vi "closed hold.vi"(2 "Acrade Drive?":bool=TRUE, 3 "Y axis value (Left)":dbl, 4 "X axis value (Right)":dbl, 5 "Threshold (.4)":dbl=0.4) -> (0 "right":dbl format="%.2f", 1 "left":dbl format="%.2f")   [LabVIEW 2014]
doc: "Holds the drivetrain position, so the robot resists movement. This is useful when balancing bridges. It's like a software brake... This VI also allows for the driver to make slight adjustments in robot position."
uses:
  <vilib>/addons/control/pid/pid.llb/PID (DBL).vi
  <vilib>/addons/control/pid/NI_PID_pid.lvlib
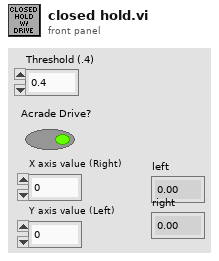
[diagram p1: front panel]
types:
  T1 = typedef "WPI_EncoderDevRef.ctl" = cluster{"DevStatus":errorcluster, "EncoderIndex":T2, "CounterIndex":T3, "DistancePerCount":dbl, "Decoding Type":T4}
  T2 = typedef "FPGA_EncoderIdx.ctl" = enum8{"Enc 0", "Enc 1", "Enc 2", "Enc 3", "Enc 4", "Enc 5", "Enc 6", "Enc 7", "Invalid"}
  T3 = typedef "FPGA_CounterCtrSystemIndex.ctl" = enum8{"Ctr 0", "Ctr 1", "Ctr 2", "Ctr 3", "Ctr 4", "Ctr 5", "Ctr 6", "Ctr 7", "Invalid"}
  T4 = typedef "WPI_EncoderType.ctl" = enum16{"1x", "2x", "4x"}
  T5 = cluster{"proportional gain (Kc)":dbl, "integral time (Ti, min)":dbl, "derivative time (Td, min)":dbl}
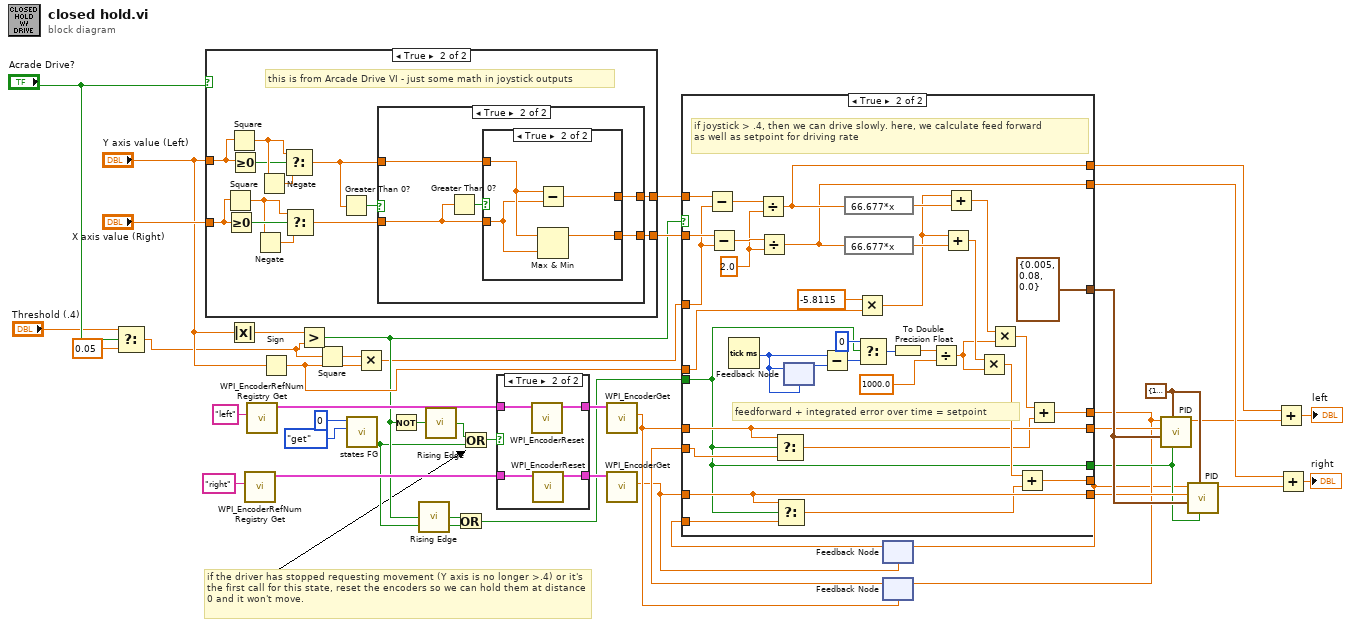
[diagram p0: block diagram]
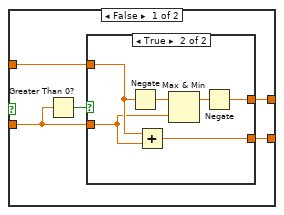
[diagram p3: hidden frame]
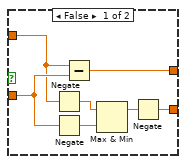
[diagram p4: hidden frame]
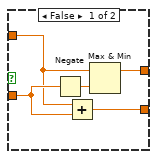
[diagram p5: hidden frame]
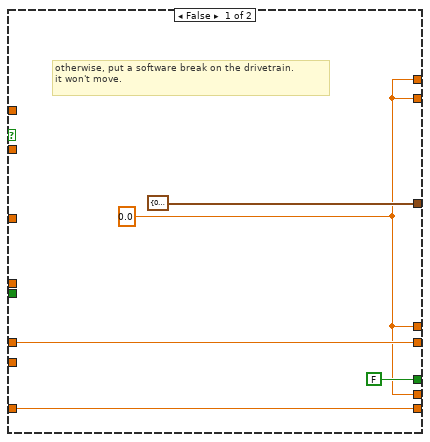
[diagram p6: hidden frame]
diagram:
  w40 = cluster{"output high":dbl, "output low":dbl} {"output high"=1.0, "output low"=-1.0} ("output range")
  # "if the driver has stopped requesting movement (Y axis is no longer >.4) or it's the first call for this state, reset the encoders so we can hold them at distance 0 and it won't move."
  n1 = Select(t="Threshold (.4)", s="Acrade Drive?", f=0.05) -> (s? t:f=w2:dbl)
  n2 = case shown="True" "Acrade Drive?" {
    tunnel: "X axis value (Right)" -> [w45 w56]
    tunnel: [w46 w49] -> w34
    tunnel: [w45 w48] -> w33
    tunnel: "Y axis value (Left)" -> [w46 w47]
    frame False {
    }
    frame True {
      # "this is from Arcade Drive VI - just some math in joystick outputs"
      n3 = Square(x=w56) -> (x^2=w54:dbl)
      n4 = Greater Or Equal To 0?(x=w56) -> (x >= 0?=w55:bool)
      n5 = Square(x=w47) -> (x^2=w51:dbl)
      n6 = Greater Or Equal To 0?(x=w47) -> (x >= 0?=w50:bool)
      n7 = Negate(x=w54) -> (-x=w53:dbl)
      n8 = Negate(x=w51) -> (-x=w52:dbl)
      n9 = Select(t=w51, s=w50, f=w52) -> (s? t:f=w58:dbl)
      n10 = Select(t=w54, s=w55, f=w53) -> (s? t:f=w57:dbl)
      n11 = Greater Than 0?(x=w58) -> (x > 0?=w59:bool)
      n12 = case shown="True" w59 {
        tunnel: w57 -> [w63 w81]
        tunnel: w58 -> [w62 w80]
        tunnel: [w61 w79] -> w49
        tunnel: [w60 w78] -> w48
        frame False {
          n13 = Greater Than 0?(x=w63) -> (x > 0?=w64:bool)
          n14 = case shown="True" w64 {
            tunnel: w63 -> [w71 w73]
            tunnel: w62 -> [w69 w74]
            tunnel: [w65 w75] -> w61
            tunnel: [w66 w72] -> w60
            frame False {
              n15 = Negate(x=w69) -> (-x=w70:dbl)
              n16 = Negate(x=w71) -> (-x=w68:dbl)
              n17 = Subtract(x=w69, y=w71) -> (x-y=w65:dbl)
              n18 = Max & Min(x=w70, y=w68) -> (max(x,y)=w67:dbl)  [unwired: 1 out]
              n19 = Negate(x=w67) -> (-x=w66:dbl)
            }
            frame True {
              n20 = Negate(x=w74) -> (-x=w77:dbl)
              n21 = Add(x=w74, y=w73) -> (x+y=w72:dbl)
              n22 = Max & Min(x=w77, y=w73) -> (max(x,y)=w76:dbl)  [unwired: 1 out]
              n23 = Negate(x=w76) -> (-x=w75:dbl)
            }
          }
        }
        frame True {
          n24 = Greater Than 0?(x=w81) -> (x > 0?=w82:bool)
          n25 = case shown="True" w82 {
            tunnel: w81 -> [w87 w89]
            tunnel: w80 -> [w84 w90]
            tunnel: [w85 w88] -> w79
            tunnel: [w83 w91] -> w78
            frame False {
              n26 = Negate(x=w87) -> (-x=w86:dbl)
              n27 = Add(x=w84, y=w87) -> (x+y=w83:dbl)
              n28 = Max & Min(x=w84, y=w86) -> (max(x,y)=w85:dbl)  [unwired: 1 out]
            }
            frame True {
              n29 = Subtract(x=w90, y=w89) -> (x-y=w88:dbl)
              n30 = Max & Min(x=w90, y=w89) -> (max(x,y)=w91:dbl)  [unwired: 1 out]
            }
          }
        }
      }
    }
  }
  n31 = Absolute Value(x="Y axis value (Left)") -> (abs(x)=w29:dbl)
  n32 = call <vilib>:"WPI_EncoderRefNum Registry Get.vi"("refnum name"="right") -> ("EncoderDevRef"=w41:T1)  [unwired: 9 in, 1 out]
  n33 = call <vilib>:"WPI_EncoderRefNum Registry Get.vi"("refnum name"="left") -> ("EncoderDevRef"=w42:T1)  [unwired: 9 in, 1 out]
  n34 = Sign(1:"Y axis value (Left)") -> (0:w22:dbl)
  n35 = Greater?(x=w29, y=w2) -> (0:w7:bool)
  n36 = Square(x=w2) -> (x^2=w8:dbl)
  n37 = call "states FG.vi"("menu (get)"=enum16{"set", "get"}."get", "Loop ID"=0) -> ("first call?"=w6:bool)  [unwired: 6 in, 3 out]
  n38 = Multiply(x=w8, y=w22) -> (x*y=w1:dbl)
  n39 = Not(x=w7) -> (.not. x?=w23:bool)
  n40 = call "Rising Edge.vi"("Input"=w7) -> ("Rising Edge"=w10:bool)
  n41 = call "Rising Edge.vi"("Input"=w23) -> ("Rising Edge"=w26:bool)
  n42 = Or(x=w10, y=w6) -> (x .or. y?=w9:bool)
  n43 = Or(x=w26, y=w6) -> (x .or. y?=w27:bool)
  n44 = case shown="True" w27 {
    tunnel: w42 -> [w93 w97]
    tunnel: w41 -> [w92 w96]
    tunnel: [w93 w95] -> w39
    tunnel: [w92 w94] -> w38
    frame False {
    }
    frame True {
      n45 = call <vilib>:"WPI_EncoderReset.vi"("EncoderDevRef"=w97) -> ("EncoderDevRef"=w95:T1)  [unwired: 9 in, 1 out]
      n46 = call <vilib>:"WPI_EncoderReset.vi"("EncoderDevRef"=w96) -> ("EncoderDevRef"=w94:T1)  [unwired: 9 in, 1 out]
    }
  }
  n47 = call <vilib>:"WPI_EncoderGet.vi"("EncoderDevRef"=w39) -> ("Distance"=w12:dbl)  [unwired: 5 in, 5 out]
  n48 = call <vilib>:"WPI_EncoderGet.vi"("EncoderDevRef"=w38) -> ("Distance"=w11:dbl)  [unwired: 5 in, 5 out]
  n49 = feedback #1(w11) -> (w14:dbl)
  n50 = feedback #2(w12) -> (w16:dbl)
  n51 = case shown="True" w7 {
    tunnel: w34 -> [_ w137]
    tunnel: w33 -> [_ w136]
    tunnel: w1 -> [_ w135]
    tunnel: [w98 w112] -> w15
    tunnel: [w98 w111] -> w13
    tunnel: [T5 {"proportional gain (Kc)"=0.08, "integral time (Ti, min)"=0.0, "derivative time (Td, min)"=0.0} ("PID gains") T5 {"proportional gain (Kc)"=0.005, "integral time (Ti, min)"=0.08, "derivative time (Td, min)"=0.0} ("PID gains")] -> w32
    tunnel: [w101 w108] -> w25
    tunnel: [w100 w105] -> w24
    tunnel: w12 -> [w101 w108]
    tunnel: w11 -> [w100 w105]
    tunnel: w22 -> [_ w127]
    tunnel: [w98 w125] -> w21
    tunnel: [w98 w124] -> w20
    tunnel: [FALSE ("Button Pressed?") w103] -> w17
    tunnel: w16 -> [_ w109]
    tunnel: w14 -> [_ w106]
    tunnel: w9 -> [_ w103]
    frame False {
      w98 = 0.0
      # "otherwise, put a software break on the drivetrain. \nit won't move."
    }
    frame True {
      w132 = 2.0 ("y")
      # "feedforward + integrated error over time = setpoint"
      # "if joystick > .4, then we can drive slowly. here, we calculate feed forward\nas well as setpoint for driving rate"
      n52 = Subtract(x=w137, y=w135) -> (x-y=w134:dbl)
      n53 = Subtract(x=w136, y=w135) -> (x-y=w133:dbl)
      n54 = Tick Count (ms)() -> (millisecond timer value=w122:u32)
      n55 = Divide(x=w134, y=w132) -> (x/y=w125:dbl)
      n56 = Divide(x=w133, y=w132) -> (x/y=w124:dbl)
      n57 = Select(t=w108, s=w103, f=w109) -> (s? t:f=w107:dbl)
      n58 = Select(t=w105, s=w103, f=w106) -> (s? t:f=w104:dbl)
      n59 = feedback-in #3(w122) -> ()
      n60 = feedback #3(w122) -> (w123:u32)
      n61 = Subtract(x=w122, y=w123) -> (x-y=w121:u32)
      n62 = expression code="66.677*x"(w125) -> (w131:dbl)
      n63 = expression code="66.677*x"(w124) -> (w130:dbl)
      n64 = Multiply(x=-5.8115 ("y"), y=w127) -> (x*y=w126:dbl)
      n65 = Select(t=u32 0, s=w103, f=w121) -> (s? t:f=w119:u32)
      n66 = To Double Precision Float(number=w119) -> (double precision float=w110:dbl)
      n67 = Divide(x=w110, y=1000.0) -> (x/y=w115:dbl)
      n68 = Add(x=w126, y=w130) -> (x+y=w116:dbl)
      n69 = Add(x=w126, y=w131) -> (x+y=w117:dbl)
      n70 = Multiply(x=w116, y=w115) -> (x*y=w113:dbl)
      n71 = Multiply(x=w117, y=w115) -> (x*y=w114:dbl)
      n72 = Add(x=w113, y=w104) -> (x+y=w111:dbl)
      n73 = Add(x=w114, y=w107) -> (x+y=w112:dbl)
    }
  }
  n74 = feedback-in #1(w13) -> ()
  n75 = feedback-in #2(w15) -> ()
  n76 = call-poly <vilib>:"PID.vi"("reinitialize? (F)"=w17, "output range"=w40, "PID gains"=w32, "process variable"=w25, "setpoint"=w15) -> ("output"=w19:dbl)  [unwired: 5 in, 1 out]
  n77 = call-poly <vilib>:"PID.vi"("reinitialize? (F)"=w17, "output range"=w40, "PID gains"=w32, "process variable"=w24, "setpoint"=w13) -> ("output"=w18:dbl)  [unwired: 5 in, 1 out]
  n78 = Add(x=w21, y=w19) -> (x+y=→"left":dbl)
  n79 = Add(x=w20, y=w18) -> (x+y=→"right":dbl)
